vi "Manipulator Stop Move.vi"(8 "error in (no error)":errorcluster, 11 "VISA resource in":refnum<visa-resource-name>="COM1") -> (0 "error out":errorcluster, 2 "Response":string, 3 "VISA resource out":refnum<visa-resource-name>)   [LabVIEW 2012, in "Scientifica Manipulator Daemon.lvlib"]
uses:
  Scientifica Manipulator Daemon.lvlib
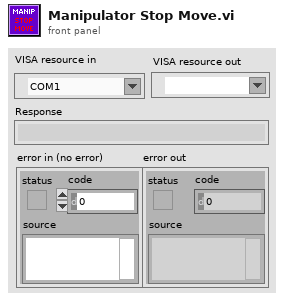
[diagram p1: front panel]
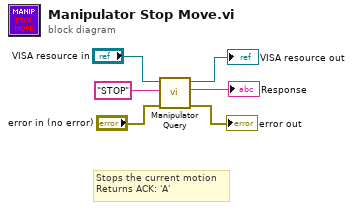
[diagram p0: block diagram]
diagram:
  # "Stops the current motion\nReturns ACK: 'A'"
  n1 = call "Manipulator Query.vi"("error in (no error)"="error in (no error)", "Command"="STOP", "VISA resource in"="VISA resource in") -> ("error out"=→"error out":errorcluster, "Response"=→"Response":string, "VISA resource out"=→"VISA resource out":refnum<visa-resource-name>)  [unwired: 5 in, 1 out]
